vi "WILT Injection Timer 1.vi"(4 "Injection Times":T1, 7 "Station Number in":u32, 8 "Error In":errorcluster, 9 "Current Threshold":dbl=1.0 format="%#_13g", 10 "Step 3 Input":T3, 11 "Dryer Step Pause In":T5 {"Night Cycle Count" format="%04d"; "Day Cycle Count" format="%04d"}) -> (0 "Error Out":errorcluster, 2 "Step 5 Output":T3, 3 "Dryer Step Pause Output":T5 {"Night Cycle Count" format="%04d"; "Day Cycle Count" format="%04d"})   [LabVIEW 2016]
uses:
  Type Definitions/WILT Station Test State Cluster.ctl
  Type Definitions/WILT Dryer Test State.ctl
  Type Definitions/WILT Dryer.ctl
  Type Definitions/WILT Dryer Details.ctl
  Type Definitions/WILT Agilent Channel Definition.ctl
  Type Definitions/WILT DAQ Data.ctl
  Type Definitions/WILT Injection Times.ctl
  Type Definitions/WILT Water Injection Control.ctl
  Globals/WILT Globals Main Program.vi
panel:
  # "Day"
  # "Night"
  # "Day"
  # "Night"
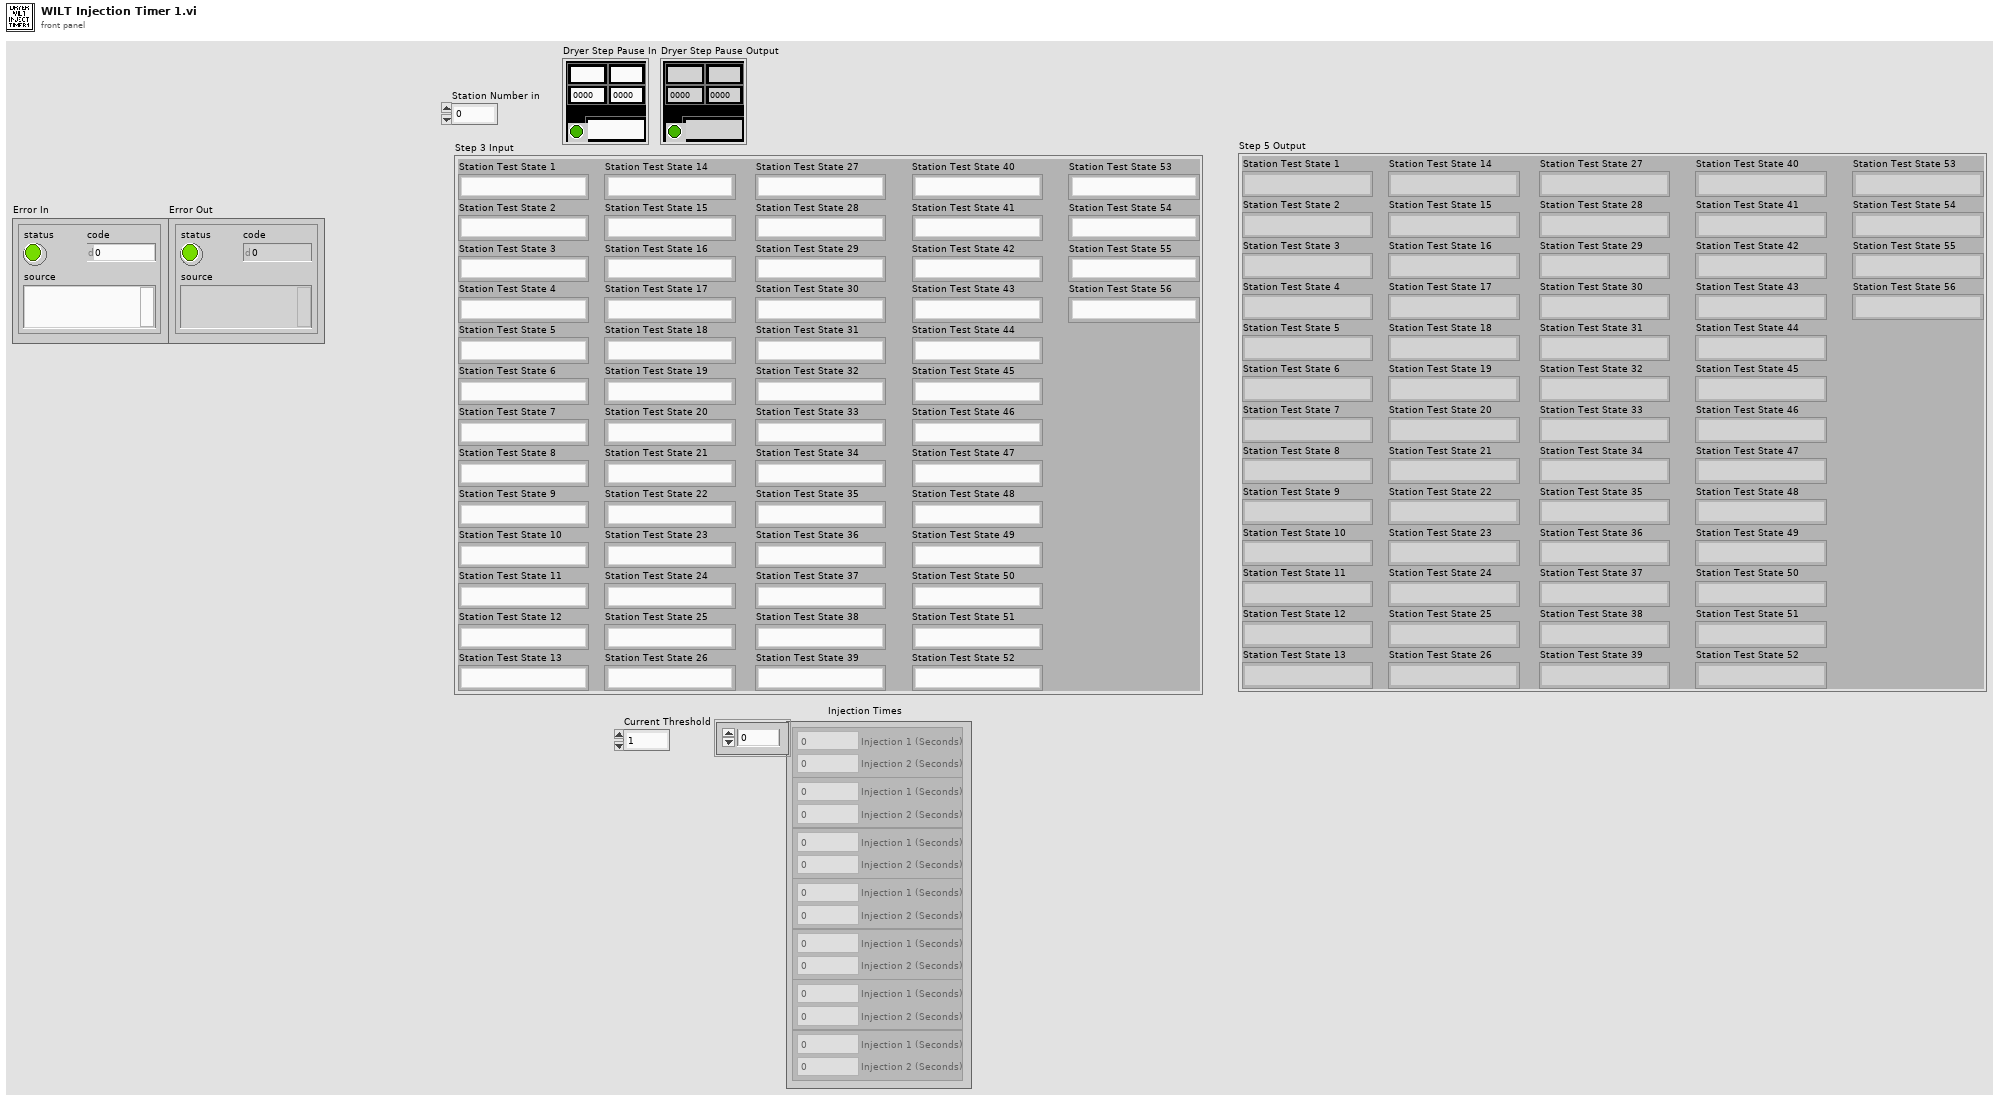
[diagram p1: front panel]
types:
  T1 = typedef "WILT Injection Times.ctl" = T2[]
  T2 = typedef "WILT Water Injection Control.ctl" = cluster{"Injection 1 (Seconds)":dbl, "Injection 2 (Seconds)":dbl}
  T3 = typedef "WILT Station Test State Cluster.ctl" = cluster{"Station Test State 1":T4, "Station Test State 2":T4, "Station Test State 3":T4, "Station Test State 4":T4, "Station Test State 5":T4, "Station Test State 6":T4, "Station Test State 7":T4, "Station Test State 8":T4, "Station Test State 9":T4, "Station Test State 10":T4, "Station Test State 11":T4, "Station Test State 12":T4, "Station Test State 13":T4, "Station Test State 14":T4, "Station Test State 15":T4, "Station Test State 16":T4, "Station Test State 17":T4, "Station Test State 18":T4, "Station Test State 19":T4, "Station Test State 20":T4, "Station Test State 21":T4, "Station Test State 22":T4, "Station Test State 23":T4, "Station Test State 24":T4, "Station Test State 25":T4, "Station Test State 26":T4, "Station Test State 27":T4, "Station Test State 28":T4, "Station Test State 29":T4, "Station Test State 30":T4, "Station Test State 31":T4, "Station Test State 32":T4, "Station Test State 33":T4, "Station Test State 34":T4, "Station Test State 35":T4, "Station Test State 36":T4, "Station Test State 37":T4, "Station Test State 38":T4, "Station Test State 39":T4, "Station Test State 40":T4, "Station Test State 41":T4, "Station Test State 42":T4, "Station Test State 43":T4, "Station Test State 44":T4, "Station Test State 45":T4, "Station Test State 46":T4, "Station Test State 47":T4, "Station Test State 48":T4, "Station Test State 49":T4, "Station Test State 50":T4, "Station Test State 51":T4, "Station Test State 52":T4, "Station Test State 53":T4, "Station Test State 54":T4, "Station Test State 55":T4, "Station Test State 56":T4}
  T4 = typedef "WILT Dryer Test State.ctl" = enum16{"No Serial Number", "Waiting for Dryer To Start", "Drying Clothes", "Water Injection 1 (On)", "Water Injection 1 Timer", "Water Injection 1 (Off)", "Pause Dryer", "Sending Start Stop CMD", "Pause Dryer 2", "Sending Start Stop CMD 2", "Drying Clothes 2", "Water Injection 2 (On)", "Water Injection 2 Timer", "Water Injection 2 (Off)", "Drying Clothes 3", "Cooling Down", "Sending Start Stop CMD 3", "Increment Cycle"}
  T5 = typedef "WILT Dryer.ctl" = cluster{"Lab ID":string, "Day Cycle Count":i32, "Station Label":string, "Dryer Details":T6, "Status Color":u32, "Invisible Button":bool, "Night Cycle Count":i32, "Station Index":i32, "Cycle Index":string, "Audit Alert":bool, "Agilent Channel Definition":T7, "DAQ Data":T8}
  T6 = typedef "WILT Dryer Details.ctl" = cluster{"Station":string, "Lab ID":string, "TR Number":string}
  T7 = typedef "WILT Agilent Channel Definition.ctl" = cluster{"Channel":string, "Station":string, "Label":string, "Agilent Station":string, "Data":dbl}
  T8 = typedef "WILT DAQ Data.ctl" = cluster{"L1 Current":dbl, "L2 Current":dbl, "Temperature  Deg F (TC)":dbl, "Volts":dbl, "Volts (208)":dbl, "SW (208)":dbl}
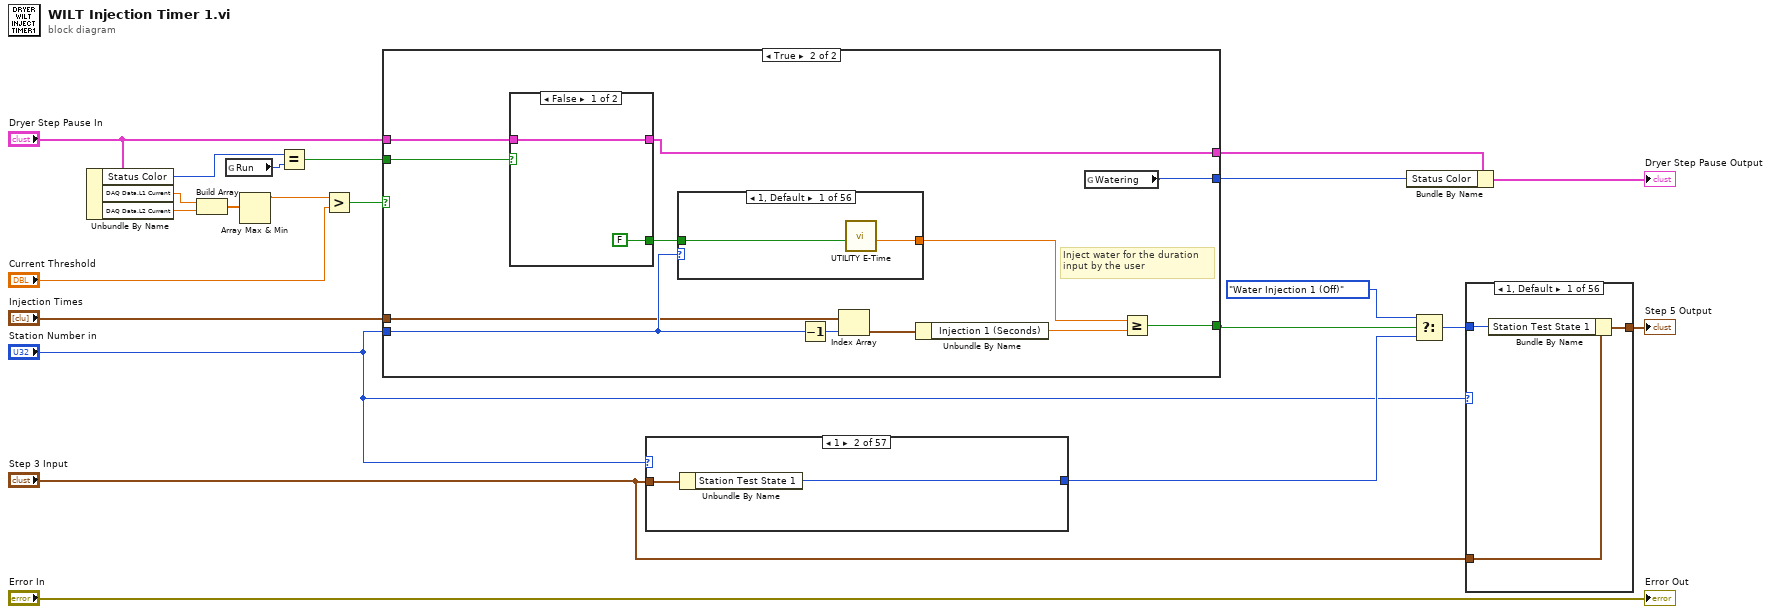
[diagram p0: block diagram]
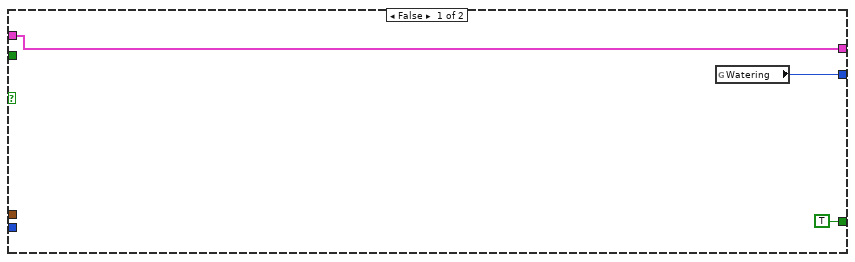
[diagram p2: hidden frame]
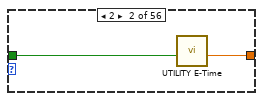
[diagram p3: hidden frame]
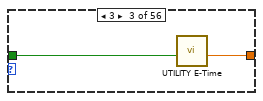
[diagram p4: hidden frame]
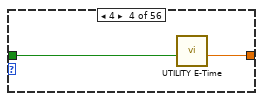
[diagram p5: hidden frame]
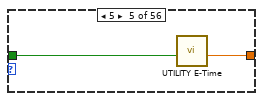
[diagram p6: hidden frame]
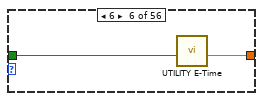
[diagram p7: hidden frame]
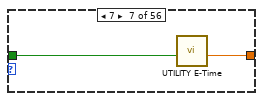
[diagram p8: hidden frame]
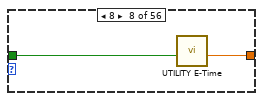
[diagram p9: hidden frame]
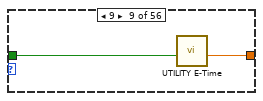
[diagram p10: hidden frame]
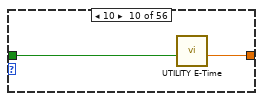
[diagram p11: hidden frame]
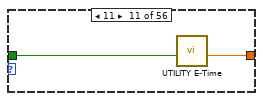
[diagram p12: hidden frame]
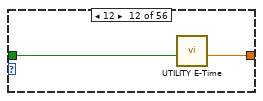
[diagram p13: hidden frame]
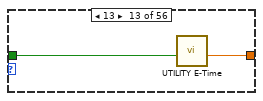
[diagram p14: hidden frame]
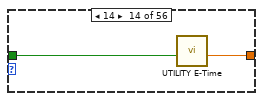
[diagram p15: hidden frame]
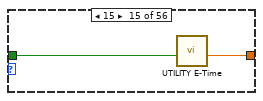
[diagram p16: hidden frame]
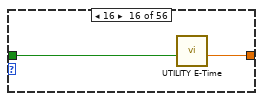
[diagram p17: hidden frame]
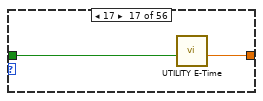
[diagram p18: hidden frame]
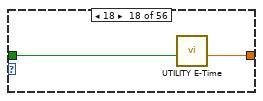
[diagram p19: hidden frame]
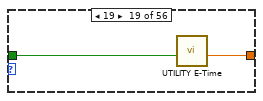
[diagram p20: hidden frame]
diagram:
  n1 = Unbundle By Name("Dryer Step Pause In") -> ("Status Color"=w15:u32, "DAQ Data.L1 Current"=w9:dbl, "DAQ Data.L2 Current"=w8:dbl)
  n2 = Build Array(w9, w8) -> (w7:dbl[])
  n3 = global read "WILT Globals Main Program.vi" "Run"() -> (w12:u32)
  n4 = Array Max & Min(array=w7) -> (max value=w5:dbl)  [unwired: 3 out]
  n5 = Equal?(x=w15, y=w12) -> (x = y?=w11:bool)
  n6 = Greater?(x=w5, y="Current Threshold") -> (0:w4:bool)
  n7 = case shown="True" w4 {
    tunnel: [TRUE w37] -> w21
    tunnel: "Dryer Step Pause In" -> [w25 w35]
    tunnel: "Station Number in" -> [_ w34]
    tunnel: w11 -> [_ w31]
    tunnel: "Injection Times" -> [_ w28]
    tunnel: [w25 w27] -> w2
    tunnel: [w23 w26] -> w1
    frame False {
      n8 = global read "WILT Globals Main Program.vi" "Watering"() -> (w23:u32)
    }
    frame True {
      # "Inject water for the duration \ninput by the user"
      n9 = case shown="False" w31 {
        tunnel: [FALSE TRUE] -> w30
        tunnel: w35 -> [w150 w152]
        tunnel: [w150 w152] -> w27
        frame False {
        }
        frame True {
        }
      }
      n10 = case shown="1, Default" w34 {
        tunnel: [w39 w40 w42 w44 w46 w48 w50 w52 w54 w56 w58 w60 w62 w64 w66 w68 w70 w72 w74 w76 w78 w80 w82 w84 w86 w88 w90 w92 w94 w96 w98 w100 w102 w104 w106 w108 w110 w112 w114 w116 w118 w120 w122 w124 w126 w128 w130 w132 w134 w136 w138 w140 w142 w144 w146 w148] -> w29
        tunnel: w30 -> [w38 w41 w43 w45 w47 w49 w51 w53 w55 w57 w59 w61 w63 w65 w67 w69 w71 w73 w75 w77 w79 w81 w83 w85 w87 w89 w91 w93 w95 w97 w99 w101 w103 w105 w107 w109 w111 w113 w115 w117 w119 w121 w123 w125 w127 w129 w131 w133 w135 w137 w139 w141 w143 w145 w147 w149]
        frame 1, Default {
          n11 = call "UTILITY E-Time.vi"("Reset"=w38) -> ("Elapsed Time (sec)"=w39:dbl)  [unwired: 8 in, 2 out]
        }
        frame 2 {
          n12 = call "UTILITY E-Time.vi"("Reset"=w41) -> ("Elapsed Time (sec)"=w40:dbl)  [unwired: 8 in, 2 out]
        }
        frame 3 {
          n13 = call "UTILITY E-Time.vi"("Reset"=w43) -> ("Elapsed Time (sec)"=w42:dbl)  [unwired: 8 in, 2 out]
        }
        frame 4 {
          n14 = call "UTILITY E-Time.vi"("Reset"=w45) -> ("Elapsed Time (sec)"=w44:dbl)  [unwired: 8 in, 2 out]
        }
        frame 5 {
          n15 = call "UTILITY E-Time.vi"("Reset"=w47) -> ("Elapsed Time (sec)"=w46:dbl)  [unwired: 8 in, 2 out]
        }
        frame 6 {
          n16 = call "UTILITY E-Time.vi"("Reset"=w49) -> ("Elapsed Time (sec)"=w48:dbl)  [unwired: 8 in, 2 out]
        }
        frame 7 {
          n17 = call "UTILITY E-Time.vi"("Reset"=w51) -> ("Elapsed Time (sec)"=w50:dbl)  [unwired: 8 in, 2 out]
        }
        frame 8 {
          n18 = call "UTILITY E-Time.vi"("Reset"=w53) -> ("Elapsed Time (sec)"=w52:dbl)  [unwired: 8 in, 2 out]
        }
        frame 9 {
          n19 = call "UTILITY E-Time.vi"("Reset"=w55) -> ("Elapsed Time (sec)"=w54:dbl)  [unwired: 8 in, 2 out]
        }
        frame 10 {
          n20 = call "UTILITY E-Time.vi"("Reset"=w57) -> ("Elapsed Time (sec)"=w56:dbl)  [unwired: 8 in, 2 out]
        }
        frame 11 {
          n21 = call "UTILITY E-Time.vi"("Reset"=w59) -> ("Elapsed Time (sec)"=w58:dbl)  [unwired: 8 in, 2 out]
        }
        frame 12 {
          n22 = call "UTILITY E-Time.vi"("Reset"=w61) -> ("Elapsed Time (sec)"=w60:dbl)  [unwired: 8 in, 2 out]
        }
        frame 13 {
          n23 = call "UTILITY E-Time.vi"("Reset"=w63) -> ("Elapsed Time (sec)"=w62:dbl)  [unwired: 8 in, 2 out]
        }
        frame 14 {
          n24 = call "UTILITY E-Time.vi"("Reset"=w65) -> ("Elapsed Time (sec)"=w64:dbl)  [unwired: 8 in, 2 out]
        }
        frame 15 {
          n25 = call "UTILITY E-Time.vi"("Reset"=w67) -> ("Elapsed Time (sec)"=w66:dbl)  [unwired: 8 in, 2 out]
        }
        frame 16 {
          n26 = call "UTILITY E-Time.vi"("Reset"=w69) -> ("Elapsed Time (sec)"=w68:dbl)  [unwired: 8 in, 2 out]
        }
        frame 17 {
          n27 = call "UTILITY E-Time.vi"("Reset"=w71) -> ("Elapsed Time (sec)"=w70:dbl)  [unwired: 8 in, 2 out]
        }
        frame 18 {
          n28 = call "UTILITY E-Time.vi"("Reset"=w73) -> ("Elapsed Time (sec)"=w72:dbl)  [unwired: 8 in, 2 out]
        }
        frame 19 {
          n29 = call "UTILITY E-Time.vi"("Reset"=w75) -> ("Elapsed Time (sec)"=w74:dbl)  [unwired: 8 in, 2 out]
        }
        frame 20 {
          n30 = call "UTILITY E-Time.vi"("Reset"=w77) -> ("Elapsed Time (sec)"=w76:dbl)  [unwired: 8 in, 2 out]
        }
        frame 21 {
          n31 = call "UTILITY E-Time.vi"("Reset"=w79) -> ("Elapsed Time (sec)"=w78:dbl)  [unwired: 8 in, 2 out]
        }
        frame 22 {
          n32 = call "UTILITY E-Time.vi"("Reset"=w81) -> ("Elapsed Time (sec)"=w80:dbl)  [unwired: 8 in, 2 out]
        }
        frame 23 {
          n33 = call "UTILITY E-Time.vi"("Reset"=w83) -> ("Elapsed Time (sec)"=w82:dbl)  [unwired: 8 in, 2 out]
        }
        frame 24 {
          n34 = call "UTILITY E-Time.vi"("Reset"=w85) -> ("Elapsed Time (sec)"=w84:dbl)  [unwired: 8 in, 2 out]
        }
        frame 25 {
          n35 = call "UTILITY E-Time.vi"("Reset"=w87) -> ("Elapsed Time (sec)"=w86:dbl)  [unwired: 8 in, 2 out]
        }
        frame 26 {
          n36 = call "UTILITY E-Time.vi"("Reset"=w89) -> ("Elapsed Time (sec)"=w88:dbl)  [unwired: 8 in, 2 out]
        }
        frame 27 {
          n37 = call "UTILITY E-Time.vi"("Reset"=w91) -> ("Elapsed Time (sec)"=w90:dbl)  [unwired: 8 in, 2 out]
        }
        frame 28 {
          n38 = call "UTILITY E-Time.vi"("Reset"=w93) -> ("Elapsed Time (sec)"=w92:dbl)  [unwired: 8 in, 2 out]
        }
        frame 29 {
          n39 = call "UTILITY E-Time.vi"("Reset"=w95) -> ("Elapsed Time (sec)"=w94:dbl)  [unwired: 8 in, 2 out]
        }
        frame 30 {
          n40 = call "UTILITY E-Time.vi"("Reset"=w97) -> ("Elapsed Time (sec)"=w96:dbl)  [unwired: 8 in, 2 out]
        }
        frame 31 {
          n41 = call "UTILITY E-Time.vi"("Reset"=w99) -> ("Elapsed Time (sec)"=w98:dbl)  [unwired: 8 in, 2 out]
        }
        frame 32 {
          n42 = call "UTILITY E-Time.vi"("Reset"=w101) -> ("Elapsed Time (sec)"=w100:dbl)  [unwired: 8 in, 2 out]
        }
        frame 33 {
          n43 = call "UTILITY E-Time.vi"("Reset"=w103) -> ("Elapsed Time (sec)"=w102:dbl)  [unwired: 8 in, 2 out]
        }
        frame 34 {
          n44 = call "UTILITY E-Time.vi"("Reset"=w105) -> ("Elapsed Time (sec)"=w104:dbl)  [unwired: 8 in, 2 out]
        }
        frame 35 {
          n45 = call "UTILITY E-Time.vi"("Reset"=w107) -> ("Elapsed Time (sec)"=w106:dbl)  [unwired: 8 in, 2 out]
        }
        frame 36 {
          n46 = call "UTILITY E-Time.vi"("Reset"=w109) -> ("Elapsed Time (sec)"=w108:dbl)  [unwired: 8 in, 2 out]
        }
        frame 37 {
          n47 = call "UTILITY E-Time.vi"("Reset"=w111) -> ("Elapsed Time (sec)"=w110:dbl)  [unwired: 8 in, 2 out]
        }
        frame 38 {
          n48 = call "UTILITY E-Time.vi"("Reset"=w113) -> ("Elapsed Time (sec)"=w112:dbl)  [unwired: 8 in, 2 out]
        }
        frame 39 {
          n49 = call "UTILITY E-Time.vi"("Reset"=w115) -> ("Elapsed Time (sec)"=w114:dbl)  [unwired: 8 in, 2 out]
        }
        frame 40 {
          n50 = call "UTILITY E-Time.vi"("Reset"=w117) -> ("Elapsed Time (sec)"=w116:dbl)  [unwired: 8 in, 2 out]
        }
        frame 41 {
          n51 = call "UTILITY E-Time.vi"("Reset"=w119) -> ("Elapsed Time (sec)"=w118:dbl)  [unwired: 8 in, 2 out]
        }
        frame 42 {
          n52 = call "UTILITY E-Time.vi"("Reset"=w121) -> ("Elapsed Time (sec)"=w120:dbl)  [unwired: 8 in, 2 out]
        }
        frame 43 {
          n53 = call "UTILITY E-Time.vi"("Reset"=w123) -> ("Elapsed Time (sec)"=w122:dbl)  [unwired: 8 in, 2 out]
        }
        frame 44 {
          n54 = call "UTILITY E-Time.vi"("Reset"=w125) -> ("Elapsed Time (sec)"=w124:dbl)  [unwired: 8 in, 2 out]
        }
        frame 45 {
          n55 = call "UTILITY E-Time.vi"("Reset"=w127) -> ("Elapsed Time (sec)"=w126:dbl)  [unwired: 8 in, 2 out]
        }
        frame 46 {
          n56 = call "UTILITY E-Time.vi"("Reset"=w129) -> ("Elapsed Time (sec)"=w128:dbl)  [unwired: 8 in, 2 out]
        }
        frame 47 {
          n57 = call "UTILITY E-Time.vi"("Reset"=w131) -> ("Elapsed Time (sec)"=w130:dbl)  [unwired: 8 in, 2 out]
        }
        frame 48 {
          n58 = call "UTILITY E-Time.vi"("Reset"=w133) -> ("Elapsed Time (sec)"=w132:dbl)  [unwired: 8 in, 2 out]
        }
        frame 49 {
          n59 = call "UTILITY E-Time.vi"("Reset"=w135) -> ("Elapsed Time (sec)"=w134:dbl)  [unwired: 8 in, 2 out]
        }
        frame 50 {
          n60 = call "UTILITY E-Time.vi"("Reset"=w137) -> ("Elapsed Time (sec)"=w136:dbl)  [unwired: 8 in, 2 out]
        }
        frame 51 {
          n61 = call "UTILITY E-Time.vi"("Reset"=w139) -> ("Elapsed Time (sec)"=w138:dbl)  [unwired: 8 in, 2 out]
        }
        frame 52 {
          n62 = call "UTILITY E-Time.vi"("Reset"=w141) -> ("Elapsed Time (sec)"=w140:dbl)  [unwired: 8 in, 2 out]
        }
        frame 53 {
          n63 = call "UTILITY E-Time.vi"("Reset"=w143) -> ("Elapsed Time (sec)"=w142:dbl)  [unwired: 8 in, 2 out]
        }
        frame 54 {
          n64 = call "UTILITY E-Time.vi"("Reset"=w145) -> ("Elapsed Time (sec)"=w144:dbl)  [unwired: 8 in, 2 out]
        }
        frame 55 {
          n65 = call "UTILITY E-Time.vi"("Reset"=w147) -> ("Elapsed Time (sec)"=w146:dbl)  [unwired: 8 in, 2 out]
        }
        frame 56 {
          n66 = call "UTILITY E-Time.vi"("Reset"=w149) -> ("Elapsed Time (sec)"=w148:dbl)  [unwired: 8 in, 2 out]
        }
      }
      n67 = Decrement(x=w34) -> (x-1=w36:u32)
      n68 = Index Array(array=w28, index=w36) -> (element=w33:T2)
      n69 = Unbundle By Name(w33) -> ("Injection 1 (Seconds)"=w32:dbl)
      n70 = global read "WILT Globals Main Program.vi" "Watering"() -> (w26:u32)
      n71 = Greater Or Equal?(x=w29, y=w32) -> (x >= y?=w37:bool)
    }
  }
  n72 = case shown="1" "Station Number in" {
    tunnel: "Step 3 Input" -> [_ w156 w158 w160 w162 w164 w166 w168 w170 w172 w174 w176 w178 w180 w182 w184 w186 w188 w190 w192 w194 w196 w198 w200 w202 w204 w206 w208 w210 w212 w214 w216 w218 w220 w222 w224 w226 w228 w230 w232 w234 w236 w238 w240 w242 w244 w246 w248 w250 w252 w254 w256 w258 w260 w262 w264 w266]
    tunnel: [WILT_Dryer_Test_State."No Serial Number" ("Station Test State 56") w155 w157 w159 w161 w163 w165 w167 w169 w171 w173 w175 w177 w179 w181 w183 w185 w187 w189 w191 w193 w195 w197 w199 w201 w203 w205 w207 w209 w211 w213 w215 w217 w219 w221 w223 w225 w227 w229 w231 w233 w235 w237 w239 w241 w243 w245 w247 w249 w251 w253 w255 w257 w259 w261 w263 w265] -> w17
    frame 0, Default {
      # "This is not a station.\nDo nothing"
    }
    frame 1 {
      n73 = Unbundle By Name(w156) -> ("Station Test State 1"=w155:T4)
    }
    frame 2 {
      n74 = Unbundle By Name(w158) -> ("Station Test State 2"=w157:T4)
    }
    frame 3 {
      n75 = Unbundle By Name(w160) -> ("Station Test State 3"=w159:T4)
    }
    frame 4 {
      n76 = Unbundle By Name(w162) -> ("Station Test State 4"=w161:T4)
    }
    frame 5 {
      n77 = Unbundle By Name(w164) -> ("Station Test State 5"=w163:T4)
    }
    frame 6 {
      n78 = Unbundle By Name(w166) -> ("Station Test State 6"=w165:T4)
    }
    frame 7 {
      n79 = Unbundle By Name(w168) -> ("Station Test State 7"=w167:T4)
    }
    frame 8 {
      n80 = Unbundle By Name(w170) -> ("Station Test State 8"=w169:T4)
    }
    frame 9 {
      n81 = Unbundle By Name(w172) -> ("Station Test State 9"=w171:T4)
    }
    frame 10 {
      n82 = Unbundle By Name(w174) -> ("Station Test State 10"=w173:T4)
    }
    frame 11 {
      n83 = Unbundle By Name(w176) -> ("Station Test State 11"=w175:T4)
    }
    frame 12 {
      n84 = Unbundle By Name(w178) -> ("Station Test State 12"=w177:T4)
    }
    frame 13 {
      n85 = Unbundle By Name(w180) -> ("Station Test State 13"=w179:T4)
    }
    frame 14 {
      n86 = Unbundle By Name(w182) -> ("Station Test State 14"=w181:T4)
    }
    frame 15 {
      n87 = Unbundle By Name(w184) -> ("Station Test State 15"=w183:T4)
    }
    frame 16 {
      n88 = Unbundle By Name(w186) -> ("Station Test State 16"=w185:T4)
    }
    frame 17 {
      n89 = Unbundle By Name(w188) -> ("Station Test State 17"=w187:T4)
    }
    frame 18 {
      n90 = Unbundle By Name(w190) -> ("Station Test State 18"=w189:T4)
    }
    frame 19 {
      n91 = Unbundle By Name(w192) -> ("Station Test State 19"=w191:T4)
    }
    frame 20 {
      n92 = Unbundle By Name(w194) -> ("Station Test State 20"=w193:T4)
    }
    frame 21 {
      n93 = Unbundle By Name(w196) -> ("Station Test State 21"=w195:T4)
    }
    frame 22 {
      n94 = Unbundle By Name(w198) -> ("Station Test State 22"=w197:T4)
    }
    frame 23 {
      n95 = Unbundle By Name(w200) -> ("Station Test State 23"=w199:T4)
    }
    frame 24 {
      n96 = Unbundle By Name(w202) -> ("Station Test State 24"=w201:T4)
    }
    frame 25 {
      n97 = Unbundle By Name(w204) -> ("Station Test State 25"=w203:T4)
    }
    frame 26 {
      n98 = Unbundle By Name(w206) -> ("Station Test State 26"=w205:T4)
    }
    frame 27 {
      n99 = Unbundle By Name(w208) -> ("Station Test State 27"=w207:T4)
    }
    frame 28 {
      n100 = Unbundle By Name(w210) -> ("Station Test State 28"=w209:T4)
    }
    frame 29 {
      n101 = Unbundle By Name(w212) -> ("Station Test State 29"=w211:T4)
    }
    frame 30 {
      n102 = Unbundle By Name(w214) -> ("Station Test State 30"=w213:T4)
    }
    frame 31 {
      n103 = Unbundle By Name(w216) -> ("Station Test State 31"=w215:T4)
    }
    frame 32 {
      n104 = Unbundle By Name(w218) -> ("Station Test State 32"=w217:T4)
    }
    frame 33 {
      n105 = Unbundle By Name(w220) -> ("Station Test State 33"=w219:T4)
    }
    frame 34 {
      n106 = Unbundle By Name(w222) -> ("Station Test State 34"=w221:T4)
    }
    frame 35 {
      n107 = Unbundle By Name(w224) -> ("Station Test State 35"=w223:T4)
    }
    frame 36 {
      n108 = Unbundle By Name(w226) -> ("Station Test State 36"=w225:T4)
    }
    frame 37 {
      n109 = Unbundle By Name(w228) -> ("Station Test State 37"=w227:T4)
    }
    frame 38 {
      n110 = Unbundle By Name(w230) -> ("Station Test State 38"=w229:T4)
    }
    frame 39 {
      n111 = Unbundle By Name(w232) -> ("Station Test State 39"=w231:T4)
    }
    frame 40 {
      n112 = Unbundle By Name(w234) -> ("Station Test State 40"=w233:T4)
    }
    frame 41 {
      n113 = Unbundle By Name(w236) -> ("Station Test State 41"=w235:T4)
    }
    frame 42 {
      n114 = Unbundle By Name(w238) -> ("Station Test State 42"=w237:T4)
    }
    frame 43 {
      n115 = Unbundle By Name(w240) -> ("Station Test State 43"=w239:T4)
    }
    frame 44 {
      n116 = Unbundle By Name(w242) -> ("Station Test State 44"=w241:T4)
    }
    frame 45 {
      n117 = Unbundle By Name(w244) -> ("Station Test State 45"=w243:T4)
    }
    frame 46 {
      n118 = Unbundle By Name(w246) -> ("Station Test State 46"=w245:T4)
    }
    frame 47 {
      n119 = Unbundle By Name(w248) -> ("Station Test State 47"=w247:T4)
    }
    frame 48 {
      n120 = Unbundle By Name(w250) -> ("Station Test State 48"=w249:T4)
    }
    frame 49 {
      n121 = Unbundle By Name(w252) -> ("Station Test State 49"=w251:T4)
    }
    frame 50 {
      n122 = Unbundle By Name(w254) -> ("Station Test State 50"=w253:T4)
    }
    frame 51 {
      n123 = Unbundle By Name(w256) -> ("Station Test State 51"=w255:T4)
    }
    frame 52 {
      n124 = Unbundle By Name(w258) -> ("Station Test State 52"=w257:T4)
    }
    frame 53 {
      n125 = Unbundle By Name(w260) -> ("Station Test State 53"=w259:T4)
    }
    frame 54 {
      n126 = Unbundle By Name(w262) -> ("Station Test State 54"=w261:T4)
    }
    frame 55 {
      n127 = Unbundle By Name(w264) -> ("Station Test State 55"=w263:T4)
    }
    frame 56 {
      n128 = Unbundle By Name(w266) -> ("Station Test State 56"=w265:T4)
    }
  }
  n129 = Bundle By Name(cluster=w2, "Status Color"=w1) -> (→"Dryer Step Pause Output":T5)
  n130 = Select(t=WILT_Dryer_Test_State."Water Injection 1 (Off)" ("Current State 2"), s=w21, f=w17) -> (s? t:f=w16:T4)
  n131 = case shown="1, Default" "Station Number in" {
    tunnel: "Step 3 Input" -> [w269 w272 w275 w278 w281 w284 w287 w290 w293 w296 w299 w302 w305 w308 w311 w314 w317 w320 w323 w326 w329 w332 w335 w338 w341 w344 w347 w350 w353 w356 w359 w362 w365 w368 w371 w374 w377 w380 w383 w386 w389 w392 w395 w398 w401 w404 w407 w410 w413 w416 w419 w422 w425 w428 w431 w434]
    tunnel: w16 -> [w268 w270 w273 w276 w279 w282 w285 w288 w291 w294 w297 w300 w303 w306 w309 w312 w315 w318 w321 w324 w327 w330 w333 w336 w339 w342 w345 w348 w351 w354 w357 w360 w363 w366 w369 w372 w375 w378 w381 w384 w387 w390 w393 w396 w399 w402 w405 w408 w411 w414 w417 w420 w423 w426 w429 w432]
    tunnel: [w267 w271 w274 w277 w280 w283 w286 w289 w292 w295 w298 w301 w304 w307 w310 w313 w316 w319 w322 w325 w328 w331 w334 w337 w340 w343 w346 w349 w352 w355 w358 w361 w364 w367 w370 w373 w376 w379 w382 w385 w388 w391 w394 w397 w400 w403 w406 w409 w412 w415 w418 w421 w424 w427 w430 w433] -> w19
    frame 1, Default {
      n132 = Bundle By Name(cluster=w269, "Station Test State 1"=w268) -> (w267:T3)
    }
    frame 2 {
      n133 = Bundle By Name(cluster=w272, "Station Test State 2"=w270) -> (w271:T3)
    }
    frame 3 {
      n134 = Bundle By Name(cluster=w275, "Station Test State 3"=w273) -> (w274:T3)
    }
    frame 4 {
      n135 = Bundle By Name(cluster=w278, "Station Test State 4"=w276) -> (w277:T3)
    }
    frame 5 {
      n136 = Bundle By Name(cluster=w281, "Station Test State 5"=w279) -> (w280:T3)
    }
    frame 6 {
      n137 = Bundle By Name(cluster=w284, "Station Test State 6"=w282) -> (w283:T3)
    }
    frame 7 {
      n138 = Bundle By Name(cluster=w287, "Station Test State 7"=w285) -> (w286:T3)
    }
    frame 8 {
      n139 = Bundle By Name(cluster=w290, "Station Test State 8"=w288) -> (w289:T3)
    }
    frame 9 {
      n140 = Bundle By Name(cluster=w293, "Station Test State 9"=w291) -> (w292:T3)
    }
    frame 10 {
      n141 = Bundle By Name(cluster=w296, "Station Test State 10"=w294) -> (w295:T3)
    }
    frame 11 {
      n142 = Bundle By Name(cluster=w299, "Station Test State 11"=w297) -> (w298:T3)
    }
    frame 12 {
      n143 = Bundle By Name(cluster=w302, "Station Test State 12"=w300) -> (w301:T3)
    }
    frame 13 {
      n144 = Bundle By Name(cluster=w305, "Station Test State 13"=w303) -> (w304:T3)
    }
    frame 14 {
      n145 = Bundle By Name(cluster=w308, "Station Test State 14"=w306) -> (w307:T3)
    }
    frame 15 {
      n146 = Bundle By Name(cluster=w311, "Station Test State 15"=w309) -> (w310:T3)
    }
    frame 16 {
      n147 = Bundle By Name(cluster=w314, "Station Test State 16"=w312) -> (w313:T3)
    }
    frame 17 {
      n148 = Bundle By Name(cluster=w317, "Station Test State 17"=w315) -> (w316:T3)
    }
    frame 18 {
      n149 = Bundle By Name(cluster=w320, "Station Test State 18"=w318) -> (w319:T3)
    }
    frame 19 {
      n150 = Bundle By Name(cluster=w323, "Station Test State 19"=w321) -> (w322:T3)
    }
    frame 20 {
      n151 = Bundle By Name(cluster=w326, "Station Test State 20"=w324) -> (w325:T3)
    }
    frame 21 {
      n152 = Bundle By Name(cluster=w329, "Station Test State 21"=w327) -> (w328:T3)
    }
    frame 22 {
      n153 = Bundle By Name(cluster=w332, "Station Test State 22"=w330) -> (w331:T3)
    }
    frame 23 {
      n154 = Bundle By Name(cluster=w335, "Station Test State 23"=w333) -> (w334:T3)
    }
    frame 24 {
      n155 = Bundle By Name(cluster=w338, "Station Test State 24"=w336) -> (w337:T3)
    }
    frame 25 {
      n156 = Bundle By Name(cluster=w341, "Station Test State 25"=w339) -> (w340:T3)
    }
    frame 26 {
      n157 = Bundle By Name(cluster=w344, "Station Test State 26"=w342) -> (w343:T3)
    }
    frame 27 {
      n158 = Bundle By Name(cluster=w347, "Station Test State 27"=w345) -> (w346:T3)
    }
    frame 28 {
      n159 = Bundle By Name(cluster=w350, "Station Test State 28"=w348) -> (w349:T3)
    }
    frame 29 {
      n160 = Bundle By Name(cluster=w353, "Station Test State 29"=w351) -> (w352:T3)
    }
    frame 30 {
      n161 = Bundle By Name(cluster=w356, "Station Test State 30"=w354) -> (w355:T3)
    }
    frame 31 {
      n162 = Bundle By Name(cluster=w359, "Station Test State 31"=w357) -> (w358:T3)
    }
    frame 32 {
      n163 = Bundle By Name(cluster=w362, "Station Test State 32"=w360) -> (w361:T3)
    }
    frame 33 {
      n164 = Bundle By Name(cluster=w365, "Station Test State 33"=w363) -> (w364:T3)
    }
    frame 34 {
      n165 = Bundle By Name(cluster=w368, "Station Test State 34"=w366) -> (w367:T3)
    }
    frame 35 {
      n166 = Bundle By Name(cluster=w371, "Station Test State 35"=w369) -> (w370:T3)
    }
    frame 36 {
      n167 = Bundle By Name(cluster=w374, "Station Test State 36"=w372) -> (w373:T3)
    }
    frame 37 {
      n168 = Bundle By Name(cluster=w377, "Station Test State 37"=w375) -> (w376:T3)
    }
    frame 38 {
      n169 = Bundle By Name(cluster=w380, "Station Test State 38"=w378) -> (w379:T3)
    }
    frame 39 {
      n170 = Bundle By Name(cluster=w383, "Station Test State 39"=w381) -> (w382:T3)
    }
    frame 40 {
      n171 = Bundle By Name(cluster=w386, "Station Test State 40"=w384) -> (w385:T3)
    }
    frame 41 {
      n172 = Bundle By Name(cluster=w389, "Station Test State 41"=w387) -> (w388:T3)
    }
    frame 42 {
      n173 = Bundle By Name(cluster=w392, "Station Test State 42"=w390) -> (w391:T3)
    }
    frame 43 {
      n174 = Bundle By Name(cluster=w395, "Station Test State 43"=w393) -> (w394:T3)
    }
    frame 44 {
      n175 = Bundle By Name(cluster=w398, "Station Test State 44"=w396) -> (w397:T3)
    }
    frame 45 {
      n176 = Bundle By Name(cluster=w401, "Station Test State 45"=w399) -> (w400:T3)
    }
    frame 46 {
      n177 = Bundle By Name(cluster=w404, "Station Test State 46"=w402) -> (w403:T3)
    }
    frame 47 {
      n178 = Bundle By Name(cluster=w407, "Station Test State 47"=w405) -> (w406:T3)
    }
    frame 48 {
      n179 = Bundle By Name(cluster=w410, "Station Test State 48"=w408) -> (w409:T3)
    }
    frame 49 {
      n180 = Bundle By Name(cluster=w413, "Station Test State 49"=w411) -> (w412:T3)
    }
    frame 50 {
      n181 = Bundle By Name(cluster=w416, "Station Test State 50"=w414) -> (w415:T3)
    }
    frame 51 {
      n182 = Bundle By Name(cluster=w419, "Station Test State 51"=w417) -> (w418:T3)
    }
    frame 52 {
      n183 = Bundle By Name(cluster=w422, "Station Test State 52"=w420) -> (w421:T3)
    }
    frame 53 {
      n184 = Bundle By Name(cluster=w425, "Station Test State 53"=w423) -> (w424:T3)
    }
    frame 54 {
      n185 = Bundle By Name(cluster=w428, "Station Test State 54"=w426) -> (w427:T3)
    }
    frame 55 {
      n186 = Bundle By Name(cluster=w431, "Station Test State 55"=w429) -> (w430:T3)
    }
    frame 56 {
      n187 = Bundle By Name(cluster=w434, "Station Test State 56"=w432) -> (w433:T3)
    }
  }
  "Step 5 Output" <- w19
  "Error Out" <- "Error In"
